vi "set_polarity_values.vi"(0 "reference (in)":i32, 2 "polarity_items":T1[](array[typedef]), 5 "error in (no error)":errorcluster) -> (14 "reference (dup)":i32, 17 "raw_value":string, 19 "error out":errorcluster)   [LabVIEW 2012]
doc: "This VI sets the Polarity settings for up to (7) items in the attached USB device. Those items are:\n\n- DIRECTION\n- LIMIT\n- HOME\n- DIGITAL OUTPUT\n- DIGITAL INPUT\n- ENABLE OUTPUT\n- JUMP TO LINE 0 ON ERROR\n\nWhen setting these values, one may choose to set all or just some of the values. For example, if one simply wants to change the logical polarity value for DIRECTION from FALSE to TRUE, the input array \"polarity_items\" would contain just one element with the 'item' set to DIRECTION and the 'value' set to TRUE. The VI does the rest!\n\nThis VI is designed to change the polarity values of ONLY those the user wishes to update (and leaves all current settings as is). \n\nProduced By:\n\nChristopher Lemieux\nKod Integrations, LLC\n4835 Marianne Drive\nMount Airy, MD 21771\nhttp://www.kodintegrations.com\nemail: clemieux@kodintegrations.com\nphone: (240) 687-1288"
uses:
  support/controls/polarity_item_group.ctl
  support/controls/polarity_items.ctl
  main_functions/commands.ctl
  support/controls/simple_actions.ctl
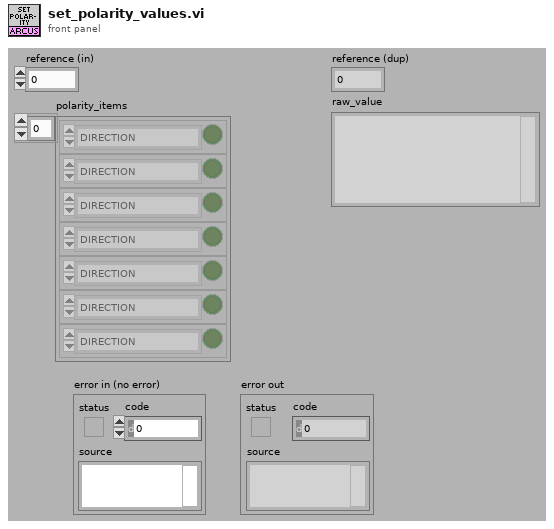
[diagram p1: front panel]
types:
  T1 = typedef "polarity_item_group.ctl" = cluster{"item":T2, "status":bool}
  T2 = typedef "polarity_items.ctl" = enum16{"DIRECTION", "LIMIT", "HOME", "DIG_OUT", "DIG_IN", "ENABLE_OUT", "JUMP_ERR"}
  T3 = typedef "simple_actions.ctl" = enum16{"from", "to"}
  T4 = typedef "commands.ctl" = enum16{"clear error", "constant jog(-)", "constant jog(+)", "get acceleration", "get actual current", "get device id", "get digital input status", "get digial inputs status", "get dig output status", "get digital outputs status", "get firmware ver", "get high speed", "get idle current", "get low speed", "get micro step", "get motor status", "get move mode", "get polarity", "get position", "get product id", "get power status", "get run current", "get status", "home(-)", "home(+)", "move to position", "power down", "power up", "set acceleration", "set device id", "set digital output", "set digital outputs", "set high speed", "set idle current", "set low speed", "set move mode absolute", "set move mode increment", "set polarity", "set position", "set run current", "stop immediate", "stop slow", "store to memory"}
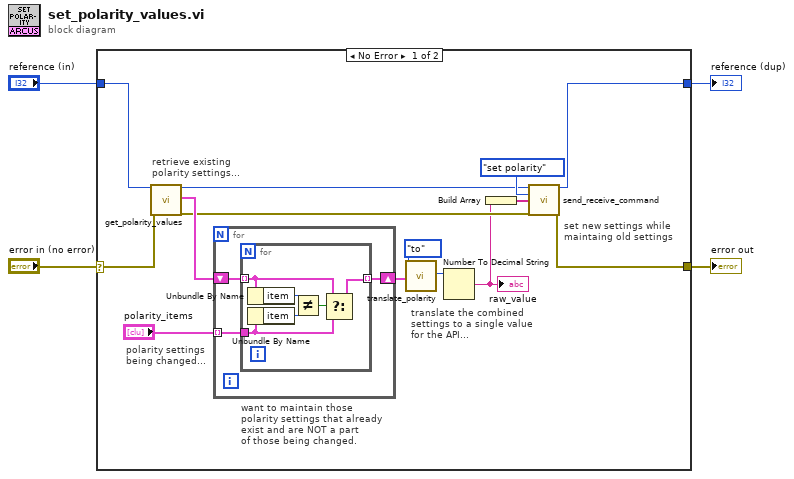
[diagram p0: block diagram]
diagram:
  n1 = case shown="No Error" "error in (no error)" {
    selector: "error in (no error)" -> [w6 w29]
    tunnel: [w18 w28] -> w4
    tunnel: [w16 w29] -> w3
    tunnel: "reference (in)" -> [w13 w28]
    frame No Error {
      # "set new settings while\nmaintaing old settings"
      # "translate the combined\nsettings to a single value\nfor the API..."
      # "polarity settings\nbeing changed..."
      # "retrieve existing\npolarity settings..."
      # "want to maintain those\npolarity settings that already\nexist and are NOT a part\nof those being changed."
      n2 = call "get_polarity_values.vi"("reference (in)"=w13, "error in (no error)"=w6) -> ("reference (dup)"=w12:i32, "polarity_items"=w10:T1[], "error out"=w9:errorcluster)  [unwired: 14 in, 1 out]
      n3 = for {
        tunnel: "polarity_items" -> [w20] mode=indexing
        shift-right: [w19] -> w8
        shift-left: w10 -> [w21]
        n4 = for {
          tunnel: w21 -> [w24] mode=indexing
          tunnel: w20 -> [w23]
          tunnel: [w22] -> w19 mode=indexing
          n5 = Unbundle By Name(w24) -> ("item"=w27:T2)
          n6 = Unbundle By Name(w23) -> ("item"=w26:T2)
          n7 = Not Equal?(x=w27, y=w26) -> (x != y?=w25:bool)
          n8 = Select(t=w24, s=w25, f=w23) -> (s? t:f=w22:T1)
        }
      }
      n9 = call "translate_polarity.vi"("simple_actions"=simple_actions."to", "polarity_items (in)"=w8) -> ("polarity_value (out)"=w14:u32)  [unwired: 16 in, 1 out]
      n10 = Number To Decimal String(number=w14) -> (decimal integer string=w5:string)  [unwired: 1 in]
      "raw_value" <- w5
      n11 = Build Array(w5) -> (w7:string[])
      n12 = call "send_receive_command.vi"("reference (in)"=w12, "command"=commands."set polarity", "params (opt)"=w7, "error in (no error)"=w9) -> ("reference (dup)"=w18:i32, "error out"=w16:errorcluster)  [unwired: 7 in, 3 out]
    }
    frame Error {
    }
  }
  "reference (dup)" <- w4
  "error out" <- w3
